vi "DBLarraytostring.vi"(11 "AI.ChanCal.Table.PreScaledVals":dbl[](array[numeric])) -> (3 "String":string)   [LabVIEW 2017]
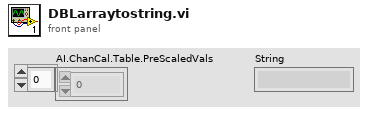
[diagram p1: front panel]
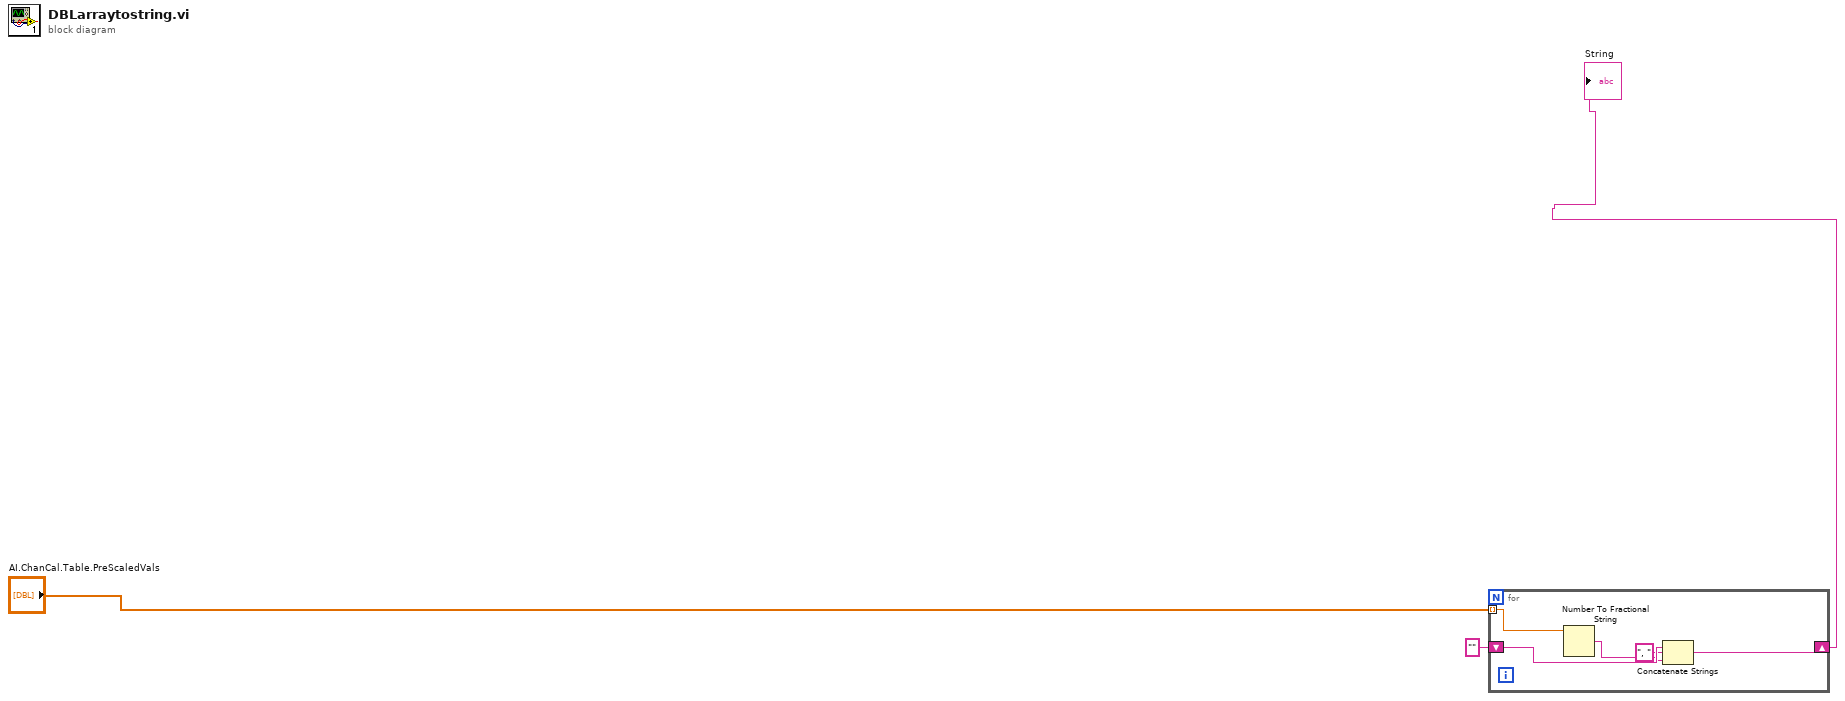
[diagram p0: block diagram]
diagram:
  n1 = for {
    tunnel: "AI.ChanCal.Table.PreScaledVals" -> [w8] mode=indexing
    shift-right: [w7] -> w3
    shift-left: "" -> [w6]
    n2 = Number To Fractional String(number=w8) -> (F-format string=w5:string)  [unwired: 3 in]
    n3 = Concatenate Strings(w6, ", " ("string"), w5) -> (w7:string)
  }
  "String" <- w3
